vi "FITS Header Rows to Table.vi"(11 "FITS Hdr Rows":T1[](array[typedef])) -> (2 "table":string[][](array[string]), 3 "Keywords":string[](array[string]))   [LabVIEW 2024]
uses:
  FITS cluster Header Row.ctl
  FITS enum Data Type.ctl
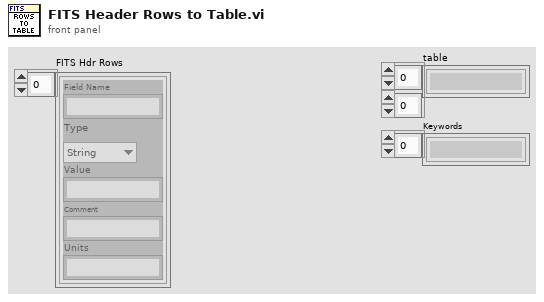
[diagram p1: front panel]
types:
  T1 = typedef "FITS cluster Header Row.ctl" = cluster{"Field Name":string, "Type":T2, "Value":string, "Comment":string, "Units":string}
  T2 = typedef "FITS enum Data Type.ctl" = enum16{"String", "Integer", "Float"}
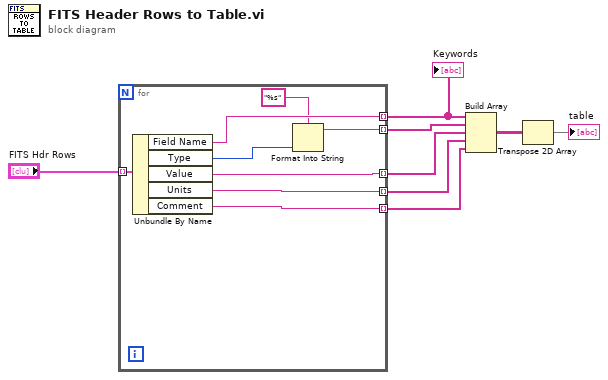
[diagram p0: block diagram]
diagram:
  n1 = for {
    tunnel: "FITS Hdr Rows" -> [w16] mode=indexing
    tunnel: [w15] -> w7 mode=indexing
    tunnel: [w10] -> w5 mode=indexing
    tunnel: [w12] -> w6 mode=indexing
    tunnel: [w11] -> w4 mode=indexing
    tunnel: [w9] -> w1 mode=indexing
    n2 = Unbundle By Name(w16) -> ("Field Name"=w15:string, "Type"=w13:T2, "Value"=w10:string, "Units"=w9:string, "Comment"=w11:string)
    n3 = Format Into String(format string="%s", w13) -> (resulting string=w12:string)  [unwired: 2 in, 1 out]
  }
  "Keywords" <- w7
  n4 = Build Array(w7, w6, w5, w1, w4) -> (w3:string[][])
  n5 = Transpose 2D Array(2D array=w3) -> (transposed array=→"table":string[][])
